vi "CheckMediatorActor.vi"(10 "Actor":refnum<class "Actor.lvclass">) -> (2 "Error":errorcluster)   [LabVIEW 2020, in "jettl.lvlib"]
uses:
  jettl.lvlib
  Actor/Actor.lvclass
  Lifetime.ctl
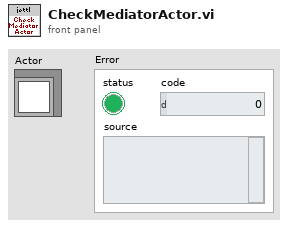
[diagram p1: front panel]
types:
  T1 = typedef "jettl.lvlib/Lifetime.ctl" = enum16{"Init", "Spawn", "Setup", "TeardownBeforeRunning", "Running", "StopCalled", "StoppingWithComponents", "StoppingNoComponents", "TeardownAfterRunning", "Stopped"}
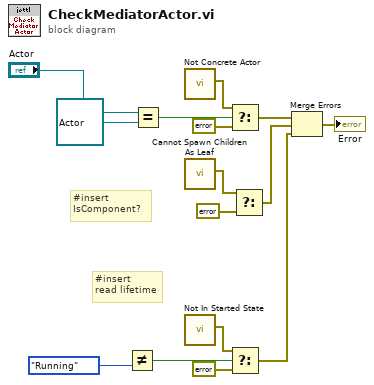
[diagram p0: block diagram]
diagram:
  # "#insert\nIsComponent?"
  # "#insert\nread lifetime"
  n1 = Not Equal?(y=Lifetime."Running") -> (x=w3:T1, x != y?=w7:bool)
  n2 = Equal?(x="Actor", y=refnum<class "Actor.lvclass"> refnum ("jettl.lvlib:Actor.lvclass")) -> (x = y?=w14:bool)
  n3 = call "Not Concrete Actor.vi"() -> ("Error"=w15:errorcluster)  [unwired: 11 in]
  n4 = call "Cannot Spawn Children As Leaf.vi"() -> ("Error"=w9:errorcluster)  [unwired: 11 in]
  n5 = call "Not In Started State.vi"() -> ("Error"=w5:errorcluster)  [unwired: 11 in]
  n6 = Select(t=w15, s=w14, f=errorcluster {"status"=FALSE, "code"=0, "source"=""}) -> (s? t:f=w13:errorcluster)
  n7 = Select(t=w5, s=w7, f=errorcluster {"status"=FALSE, "code"=0, "source"=""}) -> (s? t:f=w6:errorcluster)
  n8 = Select(t=w9, f=errorcluster {"status"=FALSE, "code"=0, "source"=""}) -> (s=w2:bool, s? t:f=w10:errorcluster)
  n9 = Merge Errors(w13, w10, w6) -> (→"Error":errorcluster)
